vi "Zapisz dane FVG.vi"(7 "Akcja (Dodaj)":T1=enum."Dodaj", 8 "error in (no error)":errorcluster, 10 "Dane":dbl, 11 "file path (use dialog)":path) -> (0 "error out":errorcluster)   [LabVIEW 2013]
uses:
  Kontrolki/FVGs/FVG save akcja.ctl
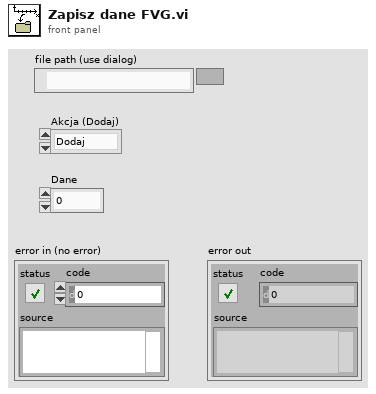
[diagram p1: front panel]
types:
  T1 = typedef "FVG save akcja.ctl" = enum16{"Wyczyœæ", "Dodaj", "Zapisz"}
  T2 = enum16{"open", "replace", "create", "open or create", "replace or create", "replace or create with confirmation"}
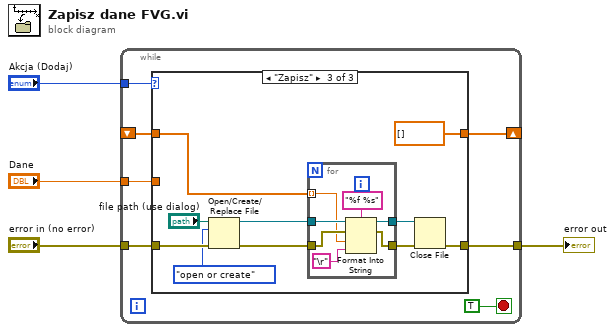
[diagram p0: block diagram]
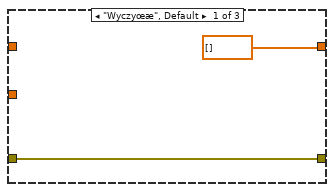
[diagram p2: hidden frame]
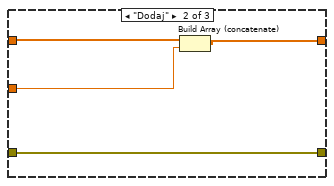
[diagram p3: hidden frame]
diagram:
  n1 = while {
    tunnel: "Akcja (Dodaj)" -> [w10]
    tunnel: "Dane" -> [w9]
    shift-right: [w8] -> _
    shift-left: _ -> [w7]
    tunnel: [w6] -> w2
    tunnel: "error in (no error)" -> [w5]
    stop <- TRUE stop-if-true
    n2 = case shown="\"Zapisz\"" w10 {
      tunnel: w9 -> [_ w17 _]
      tunnel: [dbl[] [] w16 dbl[] []] -> w8
      tunnel: w7 -> [_ w15 w19]
      tunnel: [w12 w14 w26] -> w6
      tunnel: w5 -> [w12 w14 w25]
      frame "Wyczyœæ", Default {
      }
      frame "Dodaj" {
        n3 = Build Array (concatenate)(w15, w17) -> (w16:dbl[])
      }
      frame "Zapisz" {
        n4 = Open/Create/Replace File(file path (use dialog)="file path (use dialog)", error in=w25, operation (0:open)=T2."open or create") -> (refnum out=w23:refnum<file>, error out=w22:errorcluster)  [unwired: 3 in, 1 out]
        n5 = for {
          tunnel: w23 -> [w34]
          tunnel: w22 -> [w33]
          tunnel: [w32] -> w21
          tunnel: [w31] -> w20
          tunnel: w19 -> [w29] mode=indexing
          n6 = Format Into String(format string="%f %s", initial string=w34, error in=w33, w29, "\r") -> (resulting string=w31:refnum<file>, error out=w32:errorcluster)
        }
        n7 = Close File(refnum=w20, error in=w21) -> (error out=w26:errorcluster)  [unwired: 1 out]
      }
    }
  }
  "error out" <- w2
